vi "StartExperiment.vi"(8 "error in (no error)":errorcluster, 11 "TrialBasedExperiment in":refnum<class "MatlabExperiment.lvclass">) -> (0 "error out":errorcluster, 3 "TrialBasedExperiment out":refnum<class "MatlabExperiment.lvclass">)   [LabVIEW 2014, in "AcquisitionCoreObjects.lvlib" / "MatlabExperiment.lvclass"]
uses:
  MatlabExperiment.lvclass
  TrialBasedExperimentObject/TrialBasedExperiment.lvclass
  Core SubVIs/Core SubVIs.lvlib
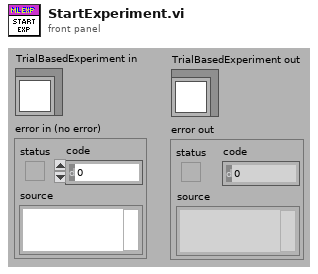
[diagram p1: front panel]
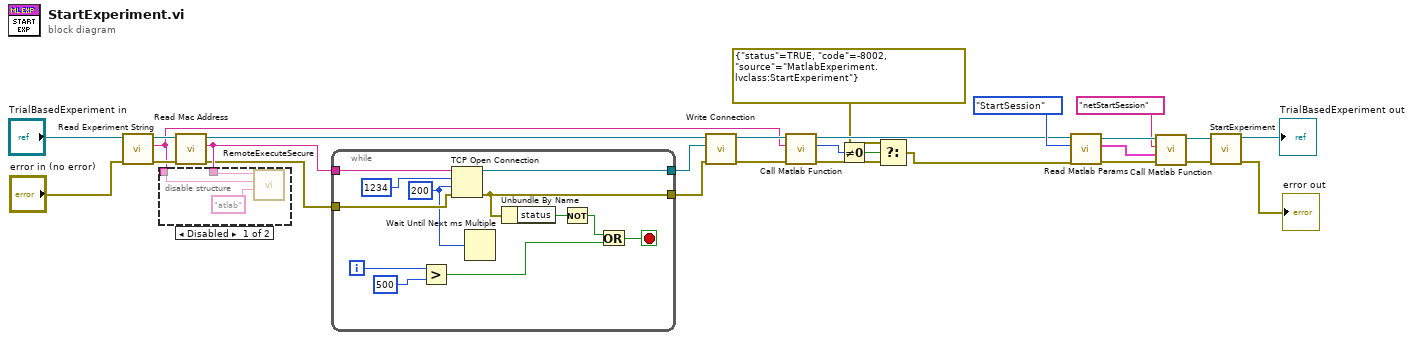
[diagram p0: block diagram]
diagram:
  n1 = call-dynamic "Read Experiment String.vi"("error in (no error)"="error in (no error)", "TrialBasedExperiment in"="TrialBasedExperiment in") -> ("error out"=w24:errorcluster, "Experiment String"=w6:string, "TrialBasedExperiment out"=w26:refnum<class "MatlabExperiment.lvclass">)  [unwired: 7 in]
  n2 = call-dynamic "Read Mac Address.vi"("error in (no error)"=w24, "TrialBasedExperiment in"=w26) -> ("error out"=w22:errorcluster, "Mac Address"=w23:string, "TrialBasedExperiment out"=w21:refnum<class "MatlabExperiment.lvclass">)  [unwired: 7 in]
  n3 = disable-structure shown="Disabled" {
    disable-tunnel: w6 -> [w30 _]
    disable-tunnel: w23 -> [w29 _]
    frame Disabled {
      n4 = call "RemoteExecuteSecure.vi"("User"="atlab", "Start Matlab Script"=w30, "IP"=w29) -> ()  [unwired: 9 out]
    }
    frame Enabled {
    }
  }
  n5 = while {
    tunnel: w23 -> [w32]
    tunnel: w22 -> [w41]
    tunnel: [w38] -> w20
    tunnel: [w33] -> w19
    i -> [w40]
    stop <- w36 stop-if-true
    w31 = 200 ("timeout ms (60000)")
    n6 = Greater?(x=w40, y=500) -> (0:w37:bool)
    n7 = TCP Open Connection(address=w32, remote port or service name=u16 1234, timeout ms (60000)=w31, error in (no error)=w41) -> (connection ID=w38:refnum<k5>, error out=w33:errorcluster)  [unwired: 1 out]
    n8 = Wait Until Next ms Multiple(millisecond multiple=w31) -> ()  [unwired: 1 out]
    n9 = Unbundle By Name(w33) -> ("status"=w34:bool)
    n10 = Not(x=w34) -> (.not. x?=w35:bool)
    n11 = Or(x=w35, y=w37) -> (x .or. y?=w36:bool)
  }
  n12 = call-dynamic "Write Connection.vi"("error in (no error)"=w19, "Connection"=w20, "TrialBasedExperiment in"=w21) -> ("error out"=w7:errorcluster, "TrialBasedExperiment out"=w9:refnum<class "MatlabExperiment.lvclass">)  [unwired: 7 in]
  n13 = call-dynamic "Call Matlab Function.vi"("error in (no error)"=w7, "Function name"=w6, "TrialBasedExperiment in"=w9) -> ("error out"=w2:errorcluster, "Return value I32"=w5:i32, "TrialBasedExperiment out"=w8:refnum<class "MatlabExperiment.lvclass">)  [unwired: 5 in, 1 out]
  n14 = Not Equal To 0?(x=w5) -> (x != 0?=w4:bool)
  n15 = Select(t=errorcluster {"status"=TRUE, "code"=-8002, "source"="MatlabExperiment.lvclass:StartExperiment"}, s=w4, f=w2) -> (s? t:f=w1:errorcluster)
  n16 = call-dynamic "Read Matlab Params.vi"("error in (no error)"=w1, "Enum"=enum16{"StartSession", "StartTrial"}."StartSession", "TrialBasedExperiment in"=w8) -> ("error out"=w14:errorcluster, "Matlab Param Array"=w11:cluster{"Name":string, "Data":variant}[], "TrialBasedExperiment out"=w13:refnum<class "MatlabExperiment.lvclass">)  [unwired: 6 in]
  n17 = call-dynamic "Call Matlab Function.vi"("error in (no error)"=w14, "Matlab Param Array"=w11, "Function name"="netStartSession", "TrialBasedExperiment in"=w13) -> ("error out"=w15:errorcluster, "TrialBasedExperiment out"=w16:refnum<class "MatlabExperiment.lvclass">)  [unwired: 4 in, 2 out]
  n18 = call-parent "StartExperiment.vi"("error in (no error)"=w15, "TrialBasedExperiment in"=w16) -> ("error out"=→"error out":errorcluster, "TrialBasedExperiment out"=→"TrialBasedExperiment out":refnum<class "MatlabExperiment.lvclass">)  [unwired: 8 in]
